vi "robust_structure_XML.vi"(0 "XML_Cluster_String":string) -> ()   [LabVIEW 2010]
uses:
  cm2nm_sample_set.ctl
  cm2nm_coordinate_information_v2.ctl
  Instrument_type_enum_v2.ctl
panel:
  out "Cluster":T1
  out "Numeric":i32
  out "output 1":i32
  out "Names":string[](array[string])
  out "Types":string[](array[string])
  out "before match":string
  out "type":string
  out "Name":string
  out "Sample Set":T2
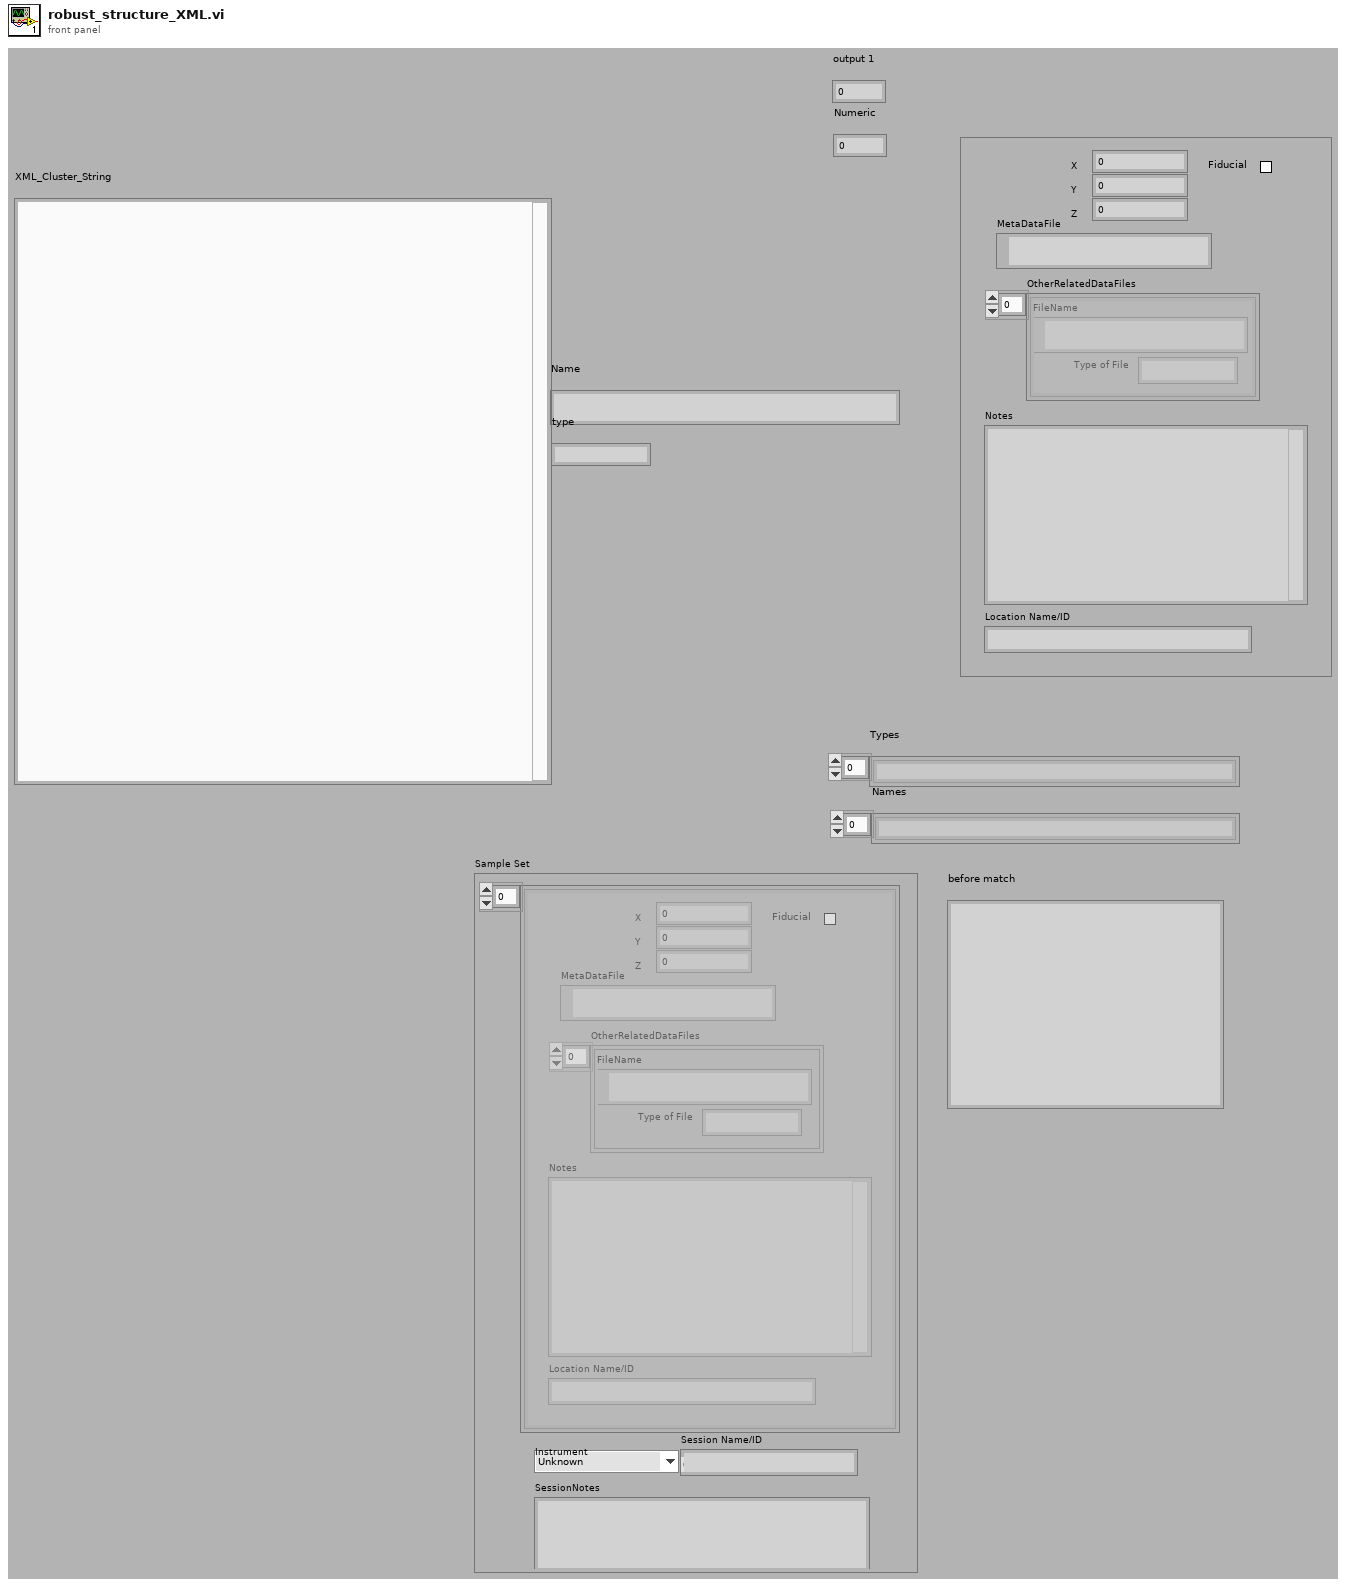
[diagram p1: front panel]
types:
  T1 = typedef "cm2nm_coordinate_information_v2.ctl" = cluster{"MetaDataFile":path, "X":dbl, "Y":dbl, "Z":dbl, "Group":i32, "Rotation":dbl[unit], "Fiducial":bool, "Magnification":dbl, "Working_Distance":dbl, "Notes":string, "Location Name/ID":string, "OtherRelatedDataFiles":cluster{"Type of File":string, "FileName":path}[], "Available":bool}
  T2 = typedef "cm2nm_sample_set.ctl" = cluster{"CollectionOfPoints":T1[], "Instrument":T3, "CollectionFile":path, "Session Name/ID":string, "SessionNotes":string}
  T3 = typedef "Instrument_type_enum_v2.ctl" = enum16{"Unknown", "Philips FEI SEM IRC", "JEOL 7000F EML_MFC", "MXRD MFC", "JEOL_EPMA"}
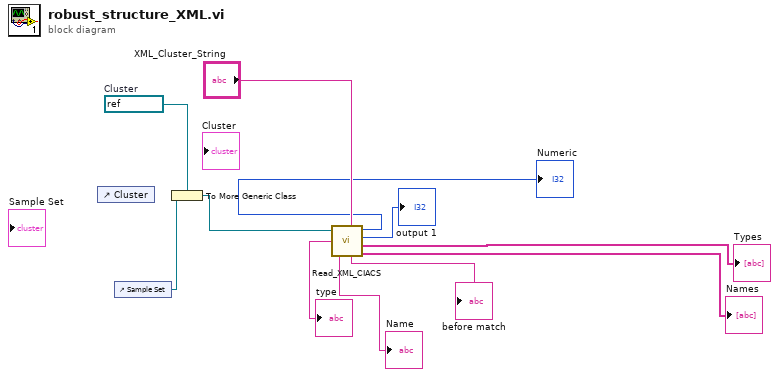
[diagram p0: block diagram]
diagram:
  w2 = refnum<vi> refnum  # Cluster
  n1 = control-ref of="Cluster"() -> ()  [unwired: 1 out]
  n2 = control-ref of="Sample Set"() -> (w1:refnum<vi>)
  n3 = To More Generic Class(target class=w2, reference=w1) -> (generic class reference=w3:refnum<vi>)
  n4 = call "Read_XML_CIACS.vi"("XML_Cluster_String"="XML_Cluster_String", "Sample Set"=w3) -> ("Numeric"=→"Numeric":i32, "output 1"=→"output 1":i32, "Array 2"=→"Types":string[], "before match"=→"before match":string, "Array"=→"Names":string[], "type"=→"type":string, "Name"=→"Name":string)
